vi "Timer.vi"(8 "error in":errorcluster, 11 "Action":enum16{"Pause", "Run", "Reset"}(ring)) -> (0 "error out":errorcluster, 3 "Time Elapsed [ms]":dbl)   [LabVIEW 2022 SP3]
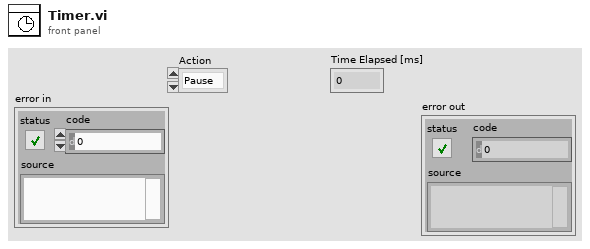
[diagram p1: front panel]
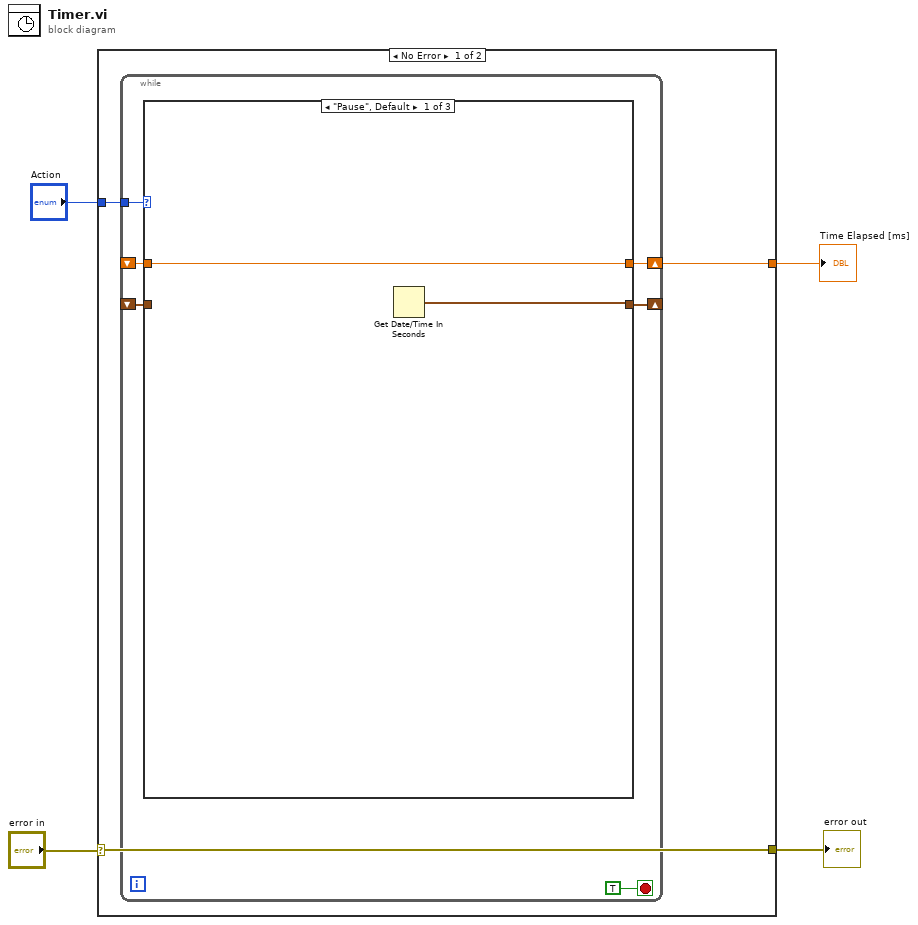
[diagram p0: block diagram]
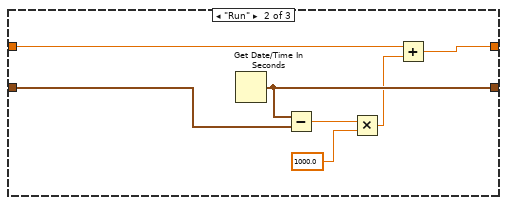
[diagram p2: hidden frame]
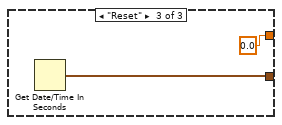
[diagram p3: hidden frame]
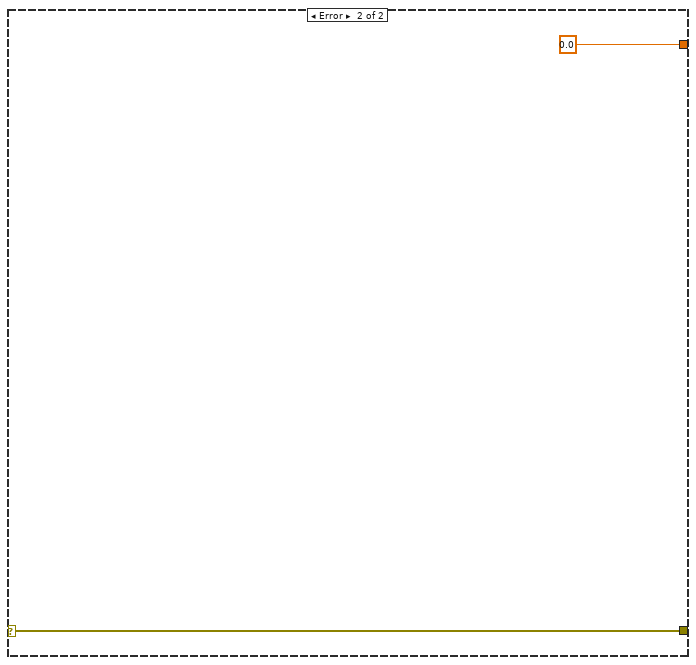
[diagram p4: hidden frame]
diagram:
  n1 = case shown="No Error" "error in" {
    selector: "error in" -> [w7 w26]
    tunnel: [w7 w26] -> w3
    tunnel: [w6 0.0] -> w2
    tunnel: "Action" -> [w5 _]
    frame No Error {
      n2 = while {
        shift-right: [w11] -> _
        shift-left: _ -> [w12]
        tunnel: w5 -> [w9]
        shift-right: [w10] -> w6
        shift-left: _ -> [w8]
        stop <- TRUE stop-if-true
        n3 = case shown="\"Pause\", Default" w9 {
          tunnel: [w15 w21 w24] -> w11
          tunnel: w12 -> [_ w22 _]
          tunnel: [w14 w20 0.0] -> w10
          tunnel: w8 -> [w14 w19 _]
          frame "Pause", Default {
            n4 = Get Date/Time In Seconds() -> (seconds since 1Jan1904=w15:timestamp)
          }
          frame "Run" {
            n5 = Get Date/Time In Seconds() -> (seconds since 1Jan1904=w21:timestamp)
            n6 = Subtract(x=w21, y=w22) -> (x-y=w18:dbl)
            n7 = Multiply(x=w18, y=1000.0) -> (x*y=w17:dbl)
            n8 = Add(x=w19, y=w17) -> (x+y=w20:dbl)
          }
          frame "Reset" {
            n9 = Get Date/Time In Seconds() -> (seconds since 1Jan1904=w24:timestamp)
          }
        }
      }
    }
    frame Error {
    }
  }
  "Time Elapsed [ms]" <- w2
  "error out" <- w3
